vi "DCC_get_mode.vi"(8 "Error In":errorcluster, 11 "DLL Path":path) -> (0 "Error Out":errorcluster, 3 "DLL Path":path)   [LabVIEW 2017]
doc: "The procedure returns the current mode of the DLL operation. Two operation modes are possible, hardware mode and simulation mode respectively.\n\nDecember 2018\nFrank Quadt & Stefan Smietana\ninfo@becker-hickl.com"
panel:
  out "Current Mode":string
  # "(c) 2021 Becker & Hickl GmbH\n     All Rights Reserved."
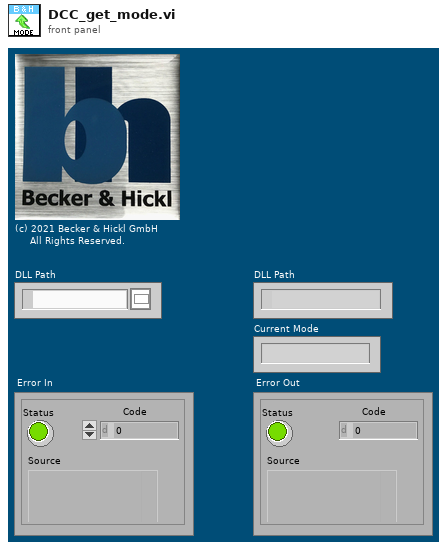
[diagram p1: front panel]
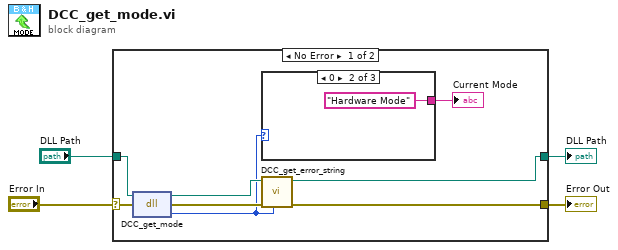
[diagram p0: block diagram]
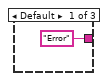
[diagram p2: hidden frame]
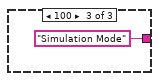
[diagram p3: hidden frame]
diagram:
  n1 = case shown="No Error" "Error In" {
    selector: "Error In" -> [w12 w17]
    tunnel: [w7 w17] -> w3
    tunnel: [w9 w16] -> w2
    tunnel: "DLL Path" -> [w10 w16]
    frame No Error {
      n2 = dll-call lib="C:/Program Files (x86)/BH/DCC/DLL/dcc64.dll" fn="DCC_get_mode"(path in=w10, error in=w12) -> (path out=w11:path, error out=w8:errorcluster, "return type"=w6:i16)  [unwired: 1 in]
      n3 = case shown="0" w6 {
        tunnel: ["Error" "Hardware Mode" "Simulation Mode"] -> w5
        frame Default {
        }
        frame 0 {
        }
        frame 100 {
        }
      }
      "Current Mode" <- w5
      n4 = call "DCC_get_error_string.vi"("Error ID"=w6, "Error In"=w8, "DLL Path"=w11) -> ("Error Out"=w7:errorcluster, "DLL Path"=w9:path)  [unwired: 6 in, 1 out]
    }
    frame Error {
    }
  }
  "Error Out" <- w3
  "DLL Path" <- w2
